vi "getServidor.vi"(11 "Cliente in":refnum<class "Cliente.lvclass">) -> (2 "servidor":string, 3 "Cliente out":refnum<class "Cliente.lvclass">)   [LabVIEW 2015, in "Cliente.lvclass"]
uses:
  Cliente.lvclass
  Cliente.lvclass/Cliente.ctl
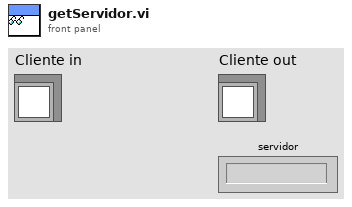
[diagram p1: front panel]
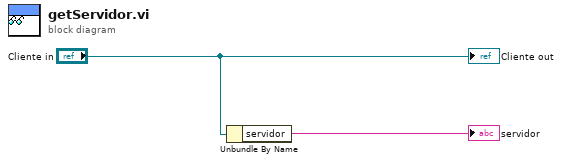
[diagram p0: block diagram]
diagram:
  n1 = Unbundle By Name("Cliente in") -> ("servidor"=→"servidor":string)
  "Cliente out" <- "Cliente in"
